vi "fan.vi"() -> ()   [LabVIEW 2020]
doc: "Manually blink and LED attached to a digital output channel of a LINX device by clicking and LED control in LabVIEW."
uses:
  <vilib>/MakerHub/LINX/Public/Peripherals/PWM/PWM Set Duty Cycle N Chans.vi
  <vilib>/MakerHub/LINX/LMH-LINX.lvlib
  <vilib>/MakerHub/LINX/Public/Peripherals/PWM/PWM Set Duty Cycle 1 Chan.vi
  <userlib>/_OpenG.lib/comparison/comparison.llb/Boolean Changed__ogtk.vi
  <vilib>/MakerHub/LINX/Public/Peripherals/Digital/Digital Write 1 Chan.vi
  <vilib>/MakerHub/LINX/Public/Utilities/Open Serial.vi
panel:
  in  "In 2":u8=4
  in  "In 1 (don't need it)":u8=3
  in  "MOTOR Channel":u8=5
  in  "Stop Button":bool
  in  "PWM Out (0-1)":dbl(knob) scale=0.0..1.0 scale format="%.2f"
  out "Loop Rate (Hz)":u32=69
  in  "DIRECTION":bool
  in  "Serial Port":refnum<visa-resource-name>="COM9"
  # "This example was created by combining code from LINX - Blink (Simple), LINX - PWM 1 Channel, and LINX - Photocell VIs\nIn addition, the circuitry for how to control a DC motor was modified from the example in:\nElegoo The Most Complete Starter Kit for UNO V2.0.2020.4.3\\English\\Part 2 Module Learning\\2.23 DC Motors"
  # "LINX Device Settings"
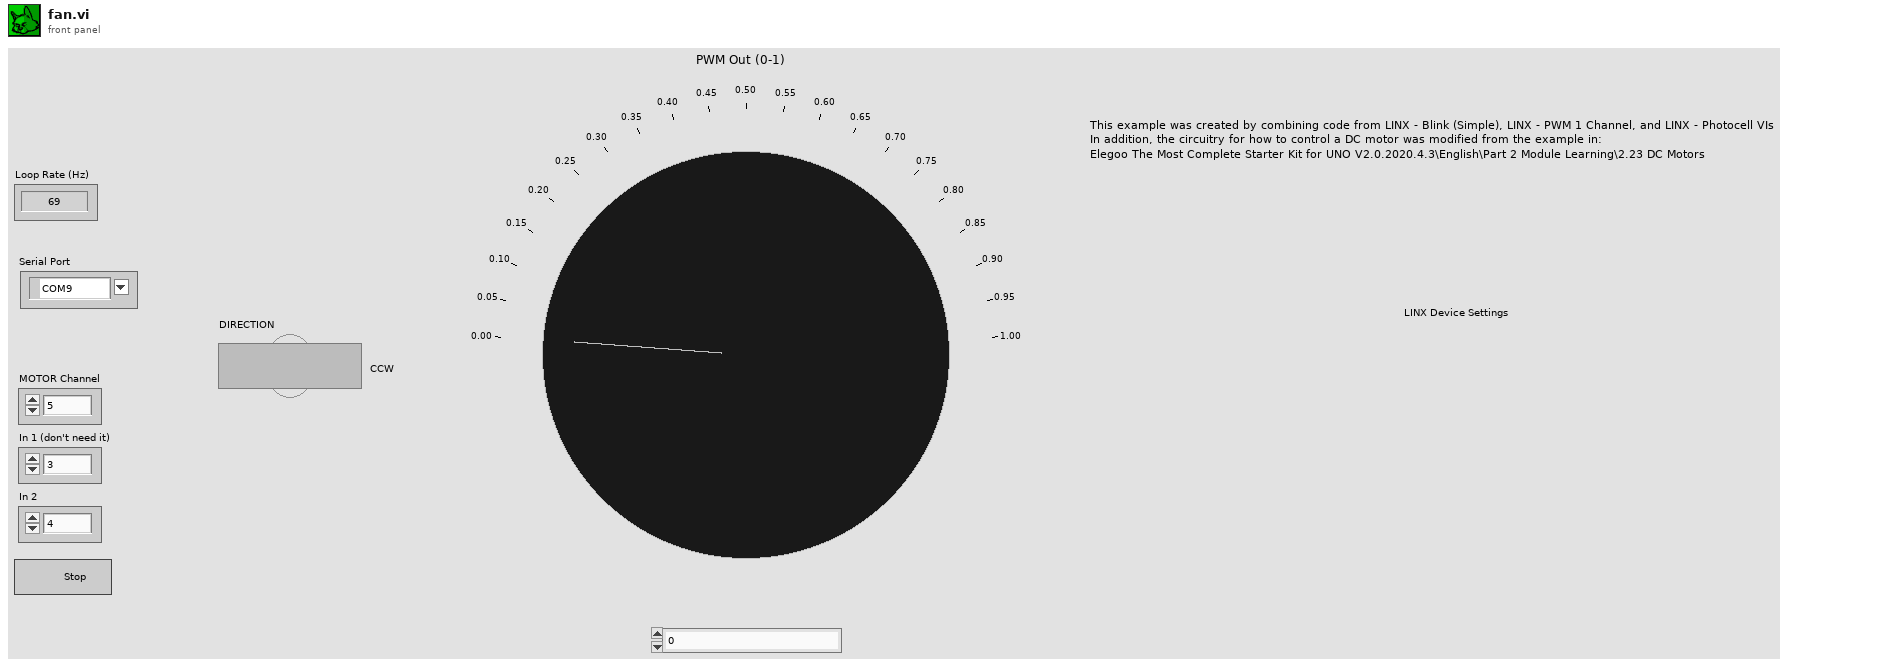
[diagram p1: front panel]
types:
  T1 = typedef "LMH-LINX.lvlib/LINX Ref.ctl" = cluster{"IO":T2, "Interface":T3, "LINX Device Config":T4}
  T2 = typedef "LMH-LINX.lvlib/Platform.ctl" = enum16{"Remote", "Local"}
  T3 = typedef "LMH-LINX.lvlib/Interface.ctl" = enum16{"Serial", "TCP"}
  T4 = typedef "LMH-LINX.lvlib/Device.lvlib/LINX Device Config.ctl" = cluster{"Interface":T3, "COM Port":refnum<visa-resource-name>, "TCP Configuration":T5, "Device Family":u8, "Device ID":u8, "Device Name":string, "TCP Ref":refnum<k5>, "Channels":T6}
  T5 = typedef "LMH-LINX.lvlib/Device.lvlib/TCP Config.ctl" = cluster{"IP Address":string, "Port":u16}
  T6 = typedef "LMH-LINX.lvlib/Channels.ctl" = cluster{"DI":u8[], "DO":u8[], "AI":u8[], "AO":u8[], "PWM":u8[], "QE":u8[], "UART":u8[], "I2C 2":u8[], "SPI":u8[], "CAN":u8[], "Servo":u8[], "AI Ref (V)":dbl, "AI Resolution (Bits)":u8, "AO Ref (V)":dbl, "AO Resolution (Bits)":u8}
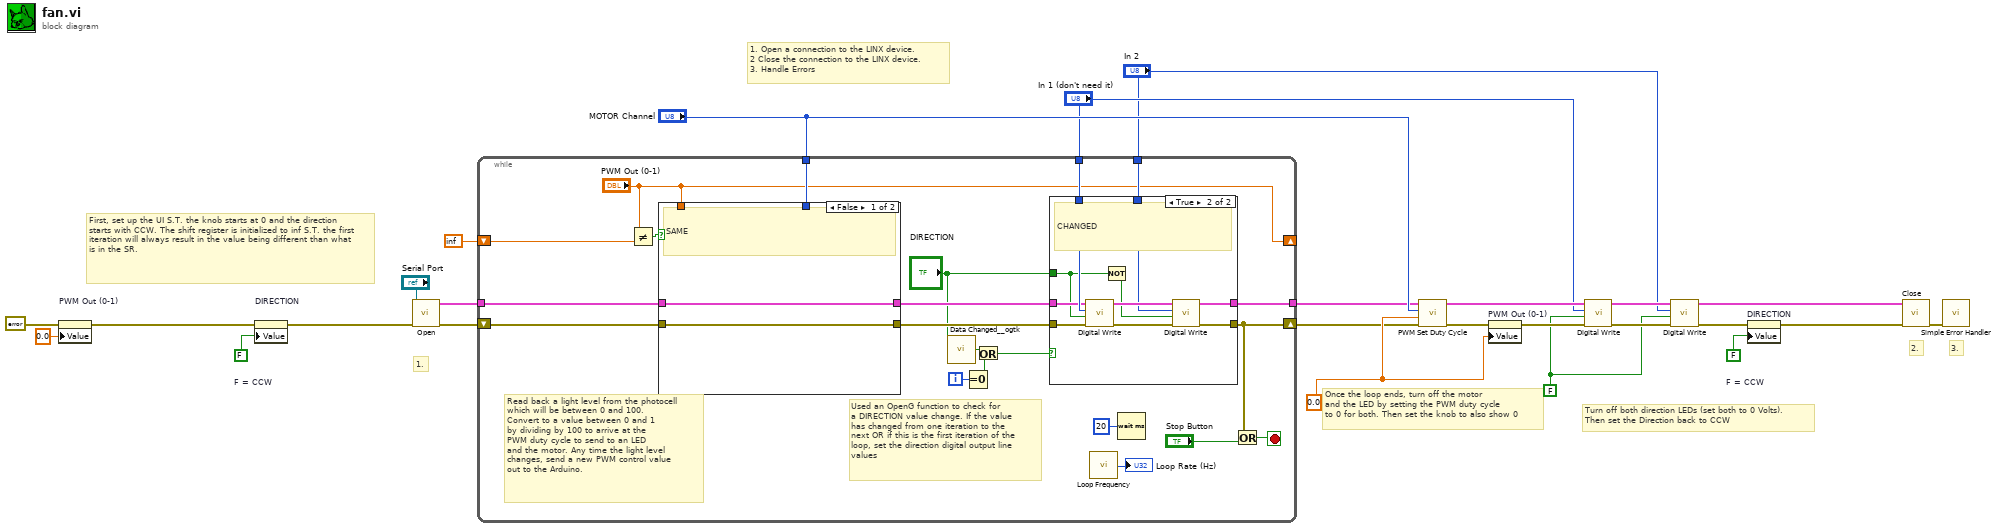
[diagram p0: block diagram]
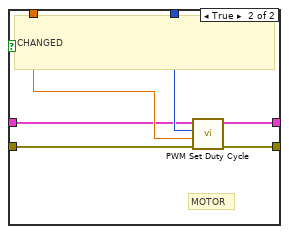
[diagram p2: hidden frame]
diagram:
  w5 = FALSE  # F = CCW
  w6 = FALSE  # F = CCW
  w9 = FALSE
  w17 = 0.0
  # "Turn off both direction LEDs (set both to 0 Volts).\nThen set the Direction back to CCW"
  # "Once the loop ends, turn off the motor\nand the LED by setting the PWM duty cycle\nto 0 for both. Then set the knob to also show 0"
  # "First, set up the UI S.T. the knob starts at 0 and the direction starts with CCW. The shift register is initialized to inf S.T. the first iteration will always result in the value being different than what is in the SR."
  # "1. Open a connection to the LINX device.\n2 Close the connection to the LINX device.\n3. Handle Errors"
  # "3."
  # "2."
  # "1."
  n1 = property on="PWM Out (0-1)" class="Knob (strict)"(error in=errorcluster {"status"=FALSE, "code"=0, "source"=""} ("Error In"), "Value"=0.0) -> (error out=w8:errorcluster)  [unwired: 1 in, 1 out]
  n2 = property on="DIRECTION" class="Bool (strict)"(error in=w8, "Value"=w6) -> (error out=w7:errorcluster)  [unwired: 1 in, 1 out]
  n3 = call-poly <vilib>:"Open.vi"("Error In"=w7, "Serial Port"="Serial Port") -> ("Error Out"=w25:errorcluster, "LINX Resource"=w26:T1)  [unwired: 7 in, 1 out]
  n4 = while {
    tunnel: w26 -> [w28]
    tunnel: [w37] -> w2
    shift-right: [w36] -> w1
    shift-left: w25 -> [w27]
    shift-right: ["PWM Out (0-1)"] -> _
    shift-left: inf -> [w44]
    tunnel: "MOTOR Channel" -> [w41]
    tunnel: "In 1 (don't need it)" -> [w40]
    tunnel: "In 2" -> [w35]
    i -> [w32]
    stop <- w47 stop-if-true
    # "Used an OpenG function to check for\na DIRECTION value change. If the value\nhas changed from one iteration to the\nnext OR if this is the first iteration of the\nloop, set the direction digital output line\nvalues"
    # "Read back a light level from the photocell\nwhich will be between 0 and 100.\nConvert to a value between 0 and 1\nby dividing by 100 to arrive at the\nPWM duty cycle to send to an LED\nand the motor. Any time the light level\nchanges, send a new PWM control value\nout to the Arduino."
    n5 = Not Equal?(x="PWM Out (0-1)", y=w44) -> (x != y?=w43:bool)
    n6 = case shown="False" w43 {
      tunnel: [w48 w55] -> w39
      tunnel: [w49 w54] -> w38
      tunnel: "PWM Out (0-1)" -> [_ w52]
      tunnel: w41 -> [_ w53]
      tunnel: w28 -> [w48 w51]
      tunnel: w27 -> [w49 w50]
      frame False {
        # "SAME"
      }
      frame True {
        # "MOTOR"
        # "CHANGED"
        n7 = call-poly <vilib>:"PWM Set Duty Cycle.vi"("Error In"=w50, "Duty Cycle (0-1)"=w52, "PWM Channel"=w53, "LINX Resource"=w51) -> ("Error Out"=w54:errorcluster, "LINX Resource"=w55:T1)  [unwired: 6 in]
      }
    }
    n8 = call-poly <userlib>:"Data Changed__ogtk.vi"("Boolean"="DIRECTION") -> ("Changed"=w29:bool)
    n9 = Equal To 0?(x=w32) -> (x = 0?=w31:bool)
    n10 = Or(x=w29, y=w31) -> (x .or. y?=w30:bool)
    n11 = case shown="True" w30 {
      tunnel: "DIRECTION" -> [_ w59]
      tunnel: w40 -> [_ w67]
      tunnel: w39 -> [w57 w66]
      tunnel: w38 -> [w56 w65]
      tunnel: [w57 w62] -> w37
      tunnel: [w56 w61] -> w36
      tunnel: w35 -> [_ w60]
      frame False {
        # "SAME"
      }
      frame True {
        # "CHANGED"
        n12 = call-poly <vilib>:"Digital Write.vi"("Error In"=w65, "Output Value"=w59, "DO Channel"=w67, "LINX Resource"=w66) -> ("Error Out"=w64:errorcluster, "LINX Resource"=w63:T1)  [unwired: 6 in]
        n13 = Not(x=w59) -> (.not. x?=w58:bool)
        n14 = call-poly <vilib>:"Digital Write.vi"("Error In"=w64, "Output Value"=w58, "DO Channel"=w60, "LINX Resource"=w63) -> ("Error Out"=w61:errorcluster, "LINX Resource"=w62:T1)  [unwired: 6 in]
      }
    }
    n15 = call <vilib>:"Loop Frequency.vi"() -> ("Loop Rate (Hz)"=→"Loop Rate (Hz)":u32)
    n16 = Wait (ms)(milliseconds to wait=u32 20) -> ()  [unwired: 1 out]
    n17 = Or(x=w36, y="Stop Button") -> (x .or. y?=w47:bool)
  }
  n18 = call-poly <vilib>:"PWM Set Duty Cycle.vi"("Error In"=w1, "Duty Cycle (0-1)"=w17, "PWM Channel"="MOTOR Channel", "LINX Resource"=w2) -> ("Error Out"=w19:errorcluster, "LINX Resource"=w16:T1)  [unwired: 6 in]
  n19 = property on="PWM Out (0-1)" class="Knob (strict)"(error in=w19, "Value"=w17) -> (error out=w12:errorcluster)  [unwired: 1 in, 1 out]
  n20 = call-poly <vilib>:"Digital Write.vi"("Error In"=w12, "Output Value"=w9, "DO Channel"="In 1 (don't need it)", "LINX Resource"=w16) -> ("Error Out"=w13:errorcluster, "LINX Resource"=w15:T1)  [unwired: 6 in]
  n21 = call-poly <vilib>:"Digital Write.vi"("Error In"=w13, "Output Value"=w9, "DO Channel"="In 2", "LINX Resource"=w15) -> ("Error Out"=w4:errorcluster, "LINX Resource"=w14:T1)  [unwired: 6 in]
  n22 = property on="DIRECTION" class="Bool (strict)"(error in=w4, "Value"=w5) -> (error out=w3:errorcluster)  [unwired: 1 in, 1 out]
  n23 = call <vilib>:"Close.vi"("Error In"=w3, "LINX Resource"=w14) -> ("Error Out"=w23:errorcluster)  [unwired: 9 in]
  n24 = call <vilib>:"Simple Error Handler.vi"("error in (no error)"=w23) -> ()  [unwired: 4 in, 5 out]
